vi "Z_Scan_v11 (SubVI).vi"(0 "Scan Axis":string, 1 "Scan Termination":T1(ring), 2 "Center of Scan":bool, 3 "Scan Type":enum16{"Sinusoidal", "Spiral"}(ring), 4 "Analog Input":i32, 5 "Table rate":i32, 6 "System no.":i32, 7 "error in (no error)":errorcluster, 8 "Z Mesh":dbl, 9 "Z-frequency":dbl, 10 "X Scan Range":dbl, 11 "Z-velocity":dbl, 12 "Z Scan Range":dbl, 14 "X Scan Center":dbl, 16 "Z Scan Center":dbl) -> (18 "3D Line Graph":refnum<class "Base Datatype.lvclass">[](array[class]), 20 "Intensity Graph":dbl[][](array[numeric]), 25 "Nano AS Data":dbl[][](array[numeric]), 26 "AS Duration (msec)":u32, 27 "error out":errorcluster)   [LabVIEW 2023]
uses:
  <vilib>/Native 3D Graph/classes/Base Datatype.lvclass
  <vilib>/Native 3D Graph/xcontrol/3DPC_SurfacePlot.xctl
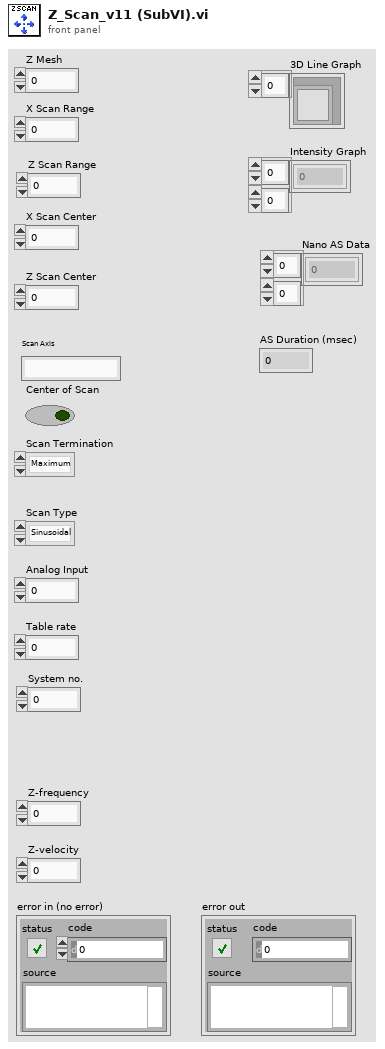
[diagram p1: front panel]
types:
  T1 = enum16{"Maximum", "End Position", "Center of scan", ""}
  T2 = cluster{"Set target type?":bool, "Target type":i32}
  T3 = cluster{"Set stop pos. option?":bool, "Stop pos. option":i32}
  T4 = cluster{"Set centroid method?":bool, "Centroid method":i32}
  T5 = cluster{"Step axis":string, "Range step axis":dbl, "Set Mid. pos?":bool, "Mid. pos. step axis":dbl}
  T6 = cluster{"Scan axis":string, "Range scan axis":dbl, "Set Mid. pos?":bool, "Mid. pos. scan axis":dbl}
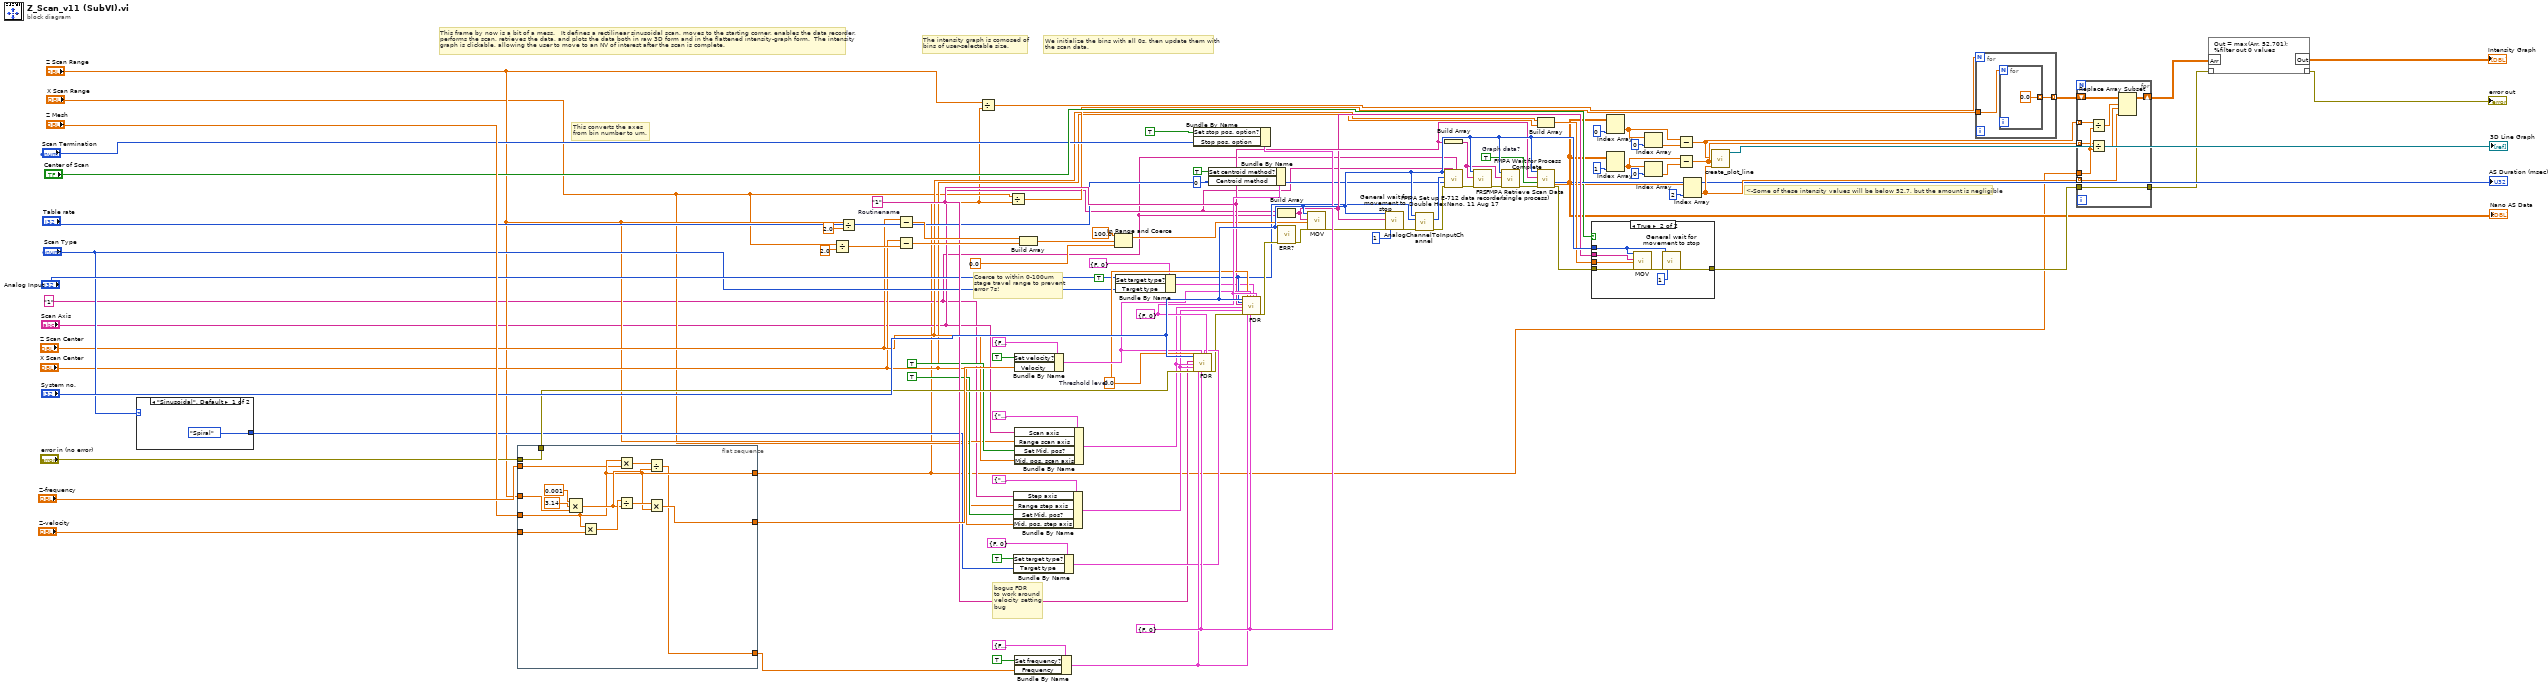
[diagram p0: block diagram]
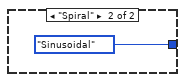
[diagram p2: hidden frame]
diagram:
  w6 = "1"
  w48 = TRUE  # Graph data?
  w81 = T3 {"Set stop pos. option?"=FALSE, "Stop pos. option"=0} ("Stop position option settings")
  w79 = T4 {"Set centroid method?"=FALSE, "Centroid method"=0} ("Centroid method settings")
  w77 = 0.0  # Threshold level
  w71 = "1"  # Routinename
  # "<-Some of these intensity values will be below 52.7, but the amount is negligible"
  # "This converts the axes\nfrom bin number to um."
  # "We initialize the bins with all 0s, then update them with\nthe scan data."
  # "The intensity graph is comosed of\nbins of user-selectable size."
  # "This frame by now is a bit of a mess.   It defines a rectilinear sinusoidal scan, moves to the starting corner, enables the data recorder,\nperforms the scan, retrieves the data, and plots the data both in raw 3D form and in the flattened intensity-graph form.  The intensity\ngraph is clickable, allowing the user to move to an NV of interest after the scan is complete."
  # "bogus FDR\nto work around\nvelocity setting\nbug"
  # "Coerce to within 0-100um\nstage travel range to prevent\nerror 7s!"
  n1 = case shown="\"Sinusoidal\", Default" "Scan Type" {
    tunnel: [enum16{"Sinusoidal", "Spiral"}."Spiral" ("Scan Type") enum16{"Sinusoidal", "Spiral"}."Sinusoidal" ("Scan Type")] -> w19
    frame "Sinusoidal", Default {
    }
    frame "Spiral" {
    }
  }
  n2 = flat-sequence {
    tunnel: "Z Scan Range" -> [w107]
    tunnel: [w103] -> w87
    tunnel: "error in (no error)" -> [w103]
    tunnel: "Z Mesh" -> [w102]
    tunnel: "Z-frequency" -> [w101]
    tunnel: "Z-velocity" -> [w100]
    tunnel: [w102] -> w3
    tunnel: [w99] -> w95
    tunnel: [w98] -> w94
    frame #0 {
      n3 = Compound Arithmetic op=MULTIPLY(0.001, 3.14, w107) -> (w105:dbl)
      n4 = Multiply(x=w102, y=w100) -> (x*y=w106:dbl)
      n5 = Multiply(x=w102, y=w101) -> (x*y=w110:dbl)
      n6 = Divide(x=w106, y=w105) -> (x/y=w104:dbl)
      n7 = Divide(x=w110, y=w105) -> (x/y=w98:dbl)
      n8 = Multiply(x=w104, y=w102) -> (x*y=w99:dbl)
    }
  }
  n9 = Divide(x="X Scan Range", y=2.0) -> (x/y=w69:dbl)
  n10 = Divide(x="Z Scan Range", y=2.0) -> (x/y=w36:dbl)
  n11 = Subtract(x="Z Scan Center", y=w36) -> (x-y=w90:dbl)
  n12 = Subtract(x="X Scan Center", y=w69) -> (x-y=w91:dbl)
  n13 = Divide(x="Z Scan Range", y=w3) -> (x/y=w13:dbl)
  n14 = Divide(x="X Scan Range", y=w3) -> (x/y=w15:dbl)
  n15 = Bundle By Name(cluster=T5 {"Step axis"="", "Range step axis"=0.1, "Set Mid. pos?"=FALSE, "Mid. pos. step axis"=0.1} ("Step axis settings"), "Step axis"=w6, "Range step axis"="X Scan Range", "Set Mid. pos?"=TRUE, "Mid. pos. step axis"="X Scan Center") -> (w72:T5)
  n16 = Bundle By Name(cluster=T2 {"Set target type?"=FALSE, "Target type"=0} ("Target type settings"), "Set target type?"=TRUE, "Target type"=w19) -> (w76:T2)
  n17 = Bundle By Name(cluster=cluster{"Set velocity?":bool, "Velocity":dbl} {"Set velocity?"=FALSE, "Velocity"=0.1} ("Velocity settings"), "Set velocity?"=TRUE ("Set target type?"), "Velocity"=w95) -> (w78:cluster{"Set velocity?":bool, "Velocity":dbl})
  n18 = Bundle By Name(cluster=T6 {"Scan axis"="", "Range scan axis"=0.1, "Set Mid. pos?"=FALSE, "Mid. pos. scan axis"=0.1} ("Scan axis settings"), "Scan axis"="Scan Axis", "Range scan axis"="Z Scan Range", "Set Mid. pos?"=TRUE, "Mid. pos. scan axis"="Z Scan Center") -> (w73:T6)
  n19 = Bundle By Name(cluster=cluster{"Set frequency?":bool, "Frequency":dbl} {"Set frequency?"=FALSE, "Frequency"=10.0} ("Frequency settings"), "Set frequency?"=TRUE, "Frequency"=w94) -> (w80:cluster{"Set frequency?":bool, "Frequency":dbl})
  n20 = Build Array(w90, w91) -> (w67:dbl[])
  n21 = In Range and Coerce(upper limit=100.0, x=w67, lower limit=0.0) -> (coerced(x)=w68:dbl[])  [unwired: 1 out]
  n22 = Bundle By Name(cluster=T2 {"Set target type?"=FALSE, "Target type"=0} ("Target type settings"), "Set target type?"=TRUE, "Target type"="Scan Type") -> (w27:T2)
  n23 = Bundle By Name(cluster=w81, "Set stop pos. option?"=TRUE, "Stop pos. option"="Scan Termination") -> ()  [unwired: 1 out]
  n24 = call "FDR.vi"("System no."="System no.", "Routinename"=w71, "Scan axis settings"=w73, "Step axis settings"=w72, "error in"=w87, "Threshold level"=w77, "Frequency settings"=w80, "Velocity settings"=w78, "Stop position option settings"=w81, "Target type settings"=w76, "Centroid method settings"=w79) -> ("error out"=w70:errorcluster)  [unwired: 3 in, 5 out]
  n25 = Bundle By Name(cluster=w79, "Set centroid method?"=TRUE, "Centroid method"=0) -> ()  [unwired: 1 out]
  n26 = call "FDR.vi"("System no."="System no.", "Board"="Analog Input", "Routinename"=w71, "Scan axis settings"=w73, "Step axis settings"=w72, "error in"=w70, "Threshold level"=w77, "Frequency settings"=w80, "Velocity settings"=w78, "Stop position option settings"=w81, "Target type settings"=w27, "Centroid method settings"=w79) -> ("error out"=w53:errorcluster)  [unwired: 2 in, 5 out]
  n27 = Build Array("Scan Axis", w6) -> (w51:string[])
  n28 = call "ERR?.vi"("System no."="System no.", "error in"=w53) -> ("error out"=w54:errorcluster)  [unwired: 16 in, 1 out]
  n29 = call "MOV.vi"("System no."="System no.", "Axes to move"=w51, "Position values"=w68, "error in"=w54) -> ("error out"=w38:errorcluster)  [unwired: 1 in, 14 out]
  n30 = call "General wait for movement to stop.vi"("System no."="System no.", "Axes to wait for"=w51, "error in"=w38, "Polling cycle \ntime, ms"=u32 1 ("Polling cycle \ntime, ms")) -> ("error out"=w39:errorcluster)  [unwired: 4 in, 11 out]
  n31 = call "AnalogChannelToInputChannel.vi"("error in (no error)"=w39, "Optical Channel In"="Analog Input", "System no."="System no.") -> ("error out"=w42:errorcluster, "Input Channel Out"=w49:i32)  [unwired: 7 in]
  n32 = Build Array(w71) -> (w47:string[])
  n33 = call "FMPA Set up E-712 data recorder - Double HexNano, 11 Aug 17.vi"("Step axis sensor ch"=w6, "Scan axis sensor ch"="Scan Axis", "error in"=w42, "Table rate"="Table rate", "Opt. Ch."=w49, "System no."="System no.") -> ("error out"=w44:errorcluster)  [unwired: 5 in]
  n34 = call "FRS.vi"("System no."="System no.", "Routines to start"=w47, "error in"=w44) -> ("error out"=w45:errorcluster)  [unwired: 16 in]
  n35 = call "FMPA Wait for Process Complete.vi"("error in"=w45, "Routines to query"=w47, "System no."="System no.") -> ("error out"=w46:errorcluster)  [unwired: 7 in, 1 out]
  n36 = Build Array("Z Scan Center", "X Scan Center") -> (w50:dbl[])
  n37 = call "FMPA Retrieve Scan Data (single process).vi"("System no."="System no.", "Process"=w71, "Graph data?"=w48, "error in"=w46) -> ("Duration (msec)"=→"AS Duration (msec)":u32, "Data"=w5:dbl[][], "error out"=w4:errorcluster)  [unwired: 10 in, 3 out]
  "Nano AS Data" <- w5
  n38 = case shown="True" "Center of Scan" {
    tunnel: w50 -> [_ w116]
    tunnel: w51 -> [_ w115]
    tunnel: w4 -> [w111 w114]
    tunnel: "System no." -> [_ w113]
    tunnel: [w111 w112] -> w20
    frame False {
    }
    frame True {
      n39 = call "MOV.vi"("System no."=w113, "Axes to move"=w115, "Position values"=w116, "error in"=w114) -> ("error out"=w118:errorcluster)  [unwired: 1 in, 14 out]
      n40 = call "General wait for movement to stop.vi"("System no."=w113, "error in"=w118, "Polling cycle \ntime, ms"=u32 1 ("Polling cycle \ntime, ms")) -> ("error out"=w112:errorcluster)  [unwired: 5 in, 11 out]
    }
  }
  n41 = Index Array(array=w5, index (col)=0 ("index")) -> (element=w58:dbl[])  [unwired: 1 in]
  n42 = Index Array(array=w5, index (col)=1 ("index")) -> (element=w55:dbl[])  [unwired: 1 in]
  n43 = Index Array(array=w58, index=0) -> (element=w59:dbl)
  n44 = Index Array(array=w55, index=0) -> (element=w56:dbl)
  n45 = Subtract(x=w58, y=w59) -> (x-y=w83:dbl[])
  n46 = Subtract(x=w55, y=w56) -> (x-y=w84:dbl[])
  n47 = Index Array(array=w5, index (col)=2 ("index")) -> (element=w85:dbl[])  [unwired: 1 in]
  n48 = call <vilib>:"create_plot_line.vi"("z vector"=w85, "y vector"=w84, "x vector"=w83) -> ("plots out"=→"3D Line Graph":refnum<class "Base Datatype.lvclass">[])  [unwired: 2 in, 6 out]
  n49 = for {
    N: w13 -> [_]
    tunnel: [w120] -> w64 mode=indexing
    tunnel: w15 -> [w119]
    n50 = for {
      N: w119 -> [_]
      tunnel: [0.0] -> w120 mode=indexing
    }
  }
  n51 = for {
    tunnel: w85 -> [w126] mode=indexing
    tunnel: w83 -> [w127] mode=indexing
    tunnel: w3 -> [w124]
    shift-right: [w128] -> w14
    shift-left: w64 -> [w125]
    tunnel: w84 -> [w123] mode=indexing
    tunnel: w20 -> [w122]
    tunnel: [w122] -> w2
    n52 = Divide(x=w127, y=w124) -> (x/y=w130:dbl)
    n53 = Divide(x=w123, y=w124) -> (x/y=w129:dbl)
    n54 = Replace Array Subset(array=w125, new element=w126, index (row)=w130, index (col)=w129) -> (w128:dbl[][])
  }
  n55 = script code="Out = max(Arr, 52.701);\n%filter out 0 values"("??"=w2, "Arr"=w14) -> ("??"=→"error out":errorcluster, "Out"=→"Intensity Graph":dbl[][])
